vi "SaveFile.vi"(9 "text":string, 11 "file path (use dialog)":path) -> ()   [LabVIEW 2017]
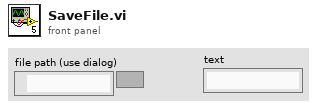
[diagram p1: front panel]
types:
  T1 = enum16{"open", "replace", "create", "open or create", "replace or create", "replace or create with confirmation"}
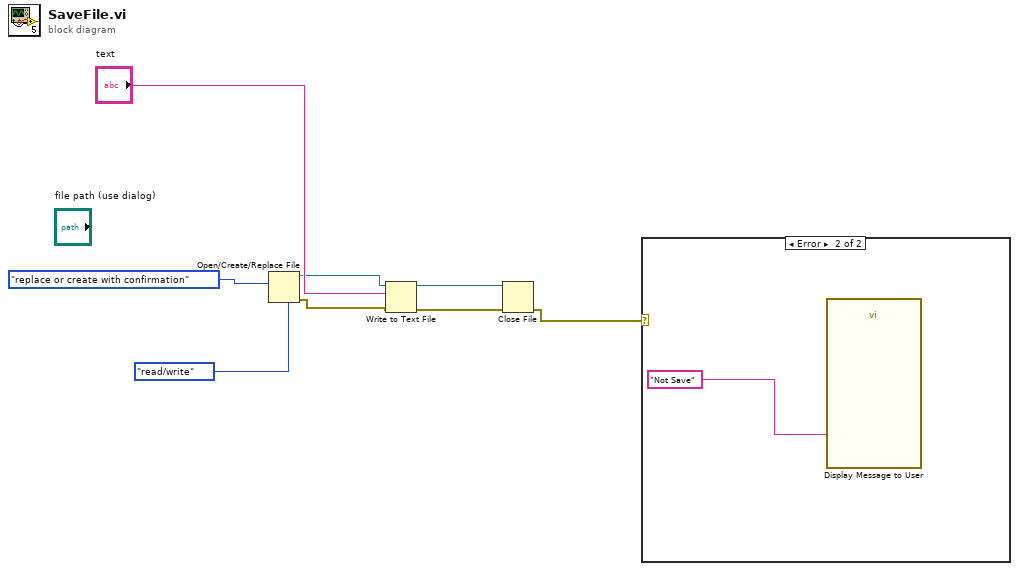
[diagram p0: block diagram]
diagram:
  n1 = Open/Create/Replace File(operation (0:open)=T1."replace or create with confirmation", access (0:read/write)=enum16{"read/write", "read-only", "write-only"}."read/write") -> (refnum out=w1:refnum<file>, error out=w5:errorcluster)  [unwired: 4 in, 1 out]
  n2 = Write to Text File(file (use dialog)=w1, text="text", error in=w5) -> (refnum out=w3:refnum<file>, error out=w4:errorcluster)  [unwired: 1 in, 1 out]
  n3 = Close File(refnum=w3, error in=w4) -> (error out=w2:errorcluster)  [unwired: 1 out]
  n4 = case shown="Error" w2 {
    frame No Error {
    }
    frame Error {
      n5 = call "Display Message to User"("Message"="Not Save") -> ()  [unwired: 9 in, 2 out]
    }
  }
